vi "ForLoopNotes.vi"() -> ()   [LabVIEW 2012]
panel:
  out "3 Loops Ago":dbl
  out "2 Loops Ago":dbl
  out "End Value":dbl
  out "New Value":dbl
  out "1 Loop Ago":dbl
  out "i":dbl
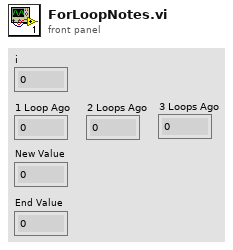
[diagram p1: front panel]
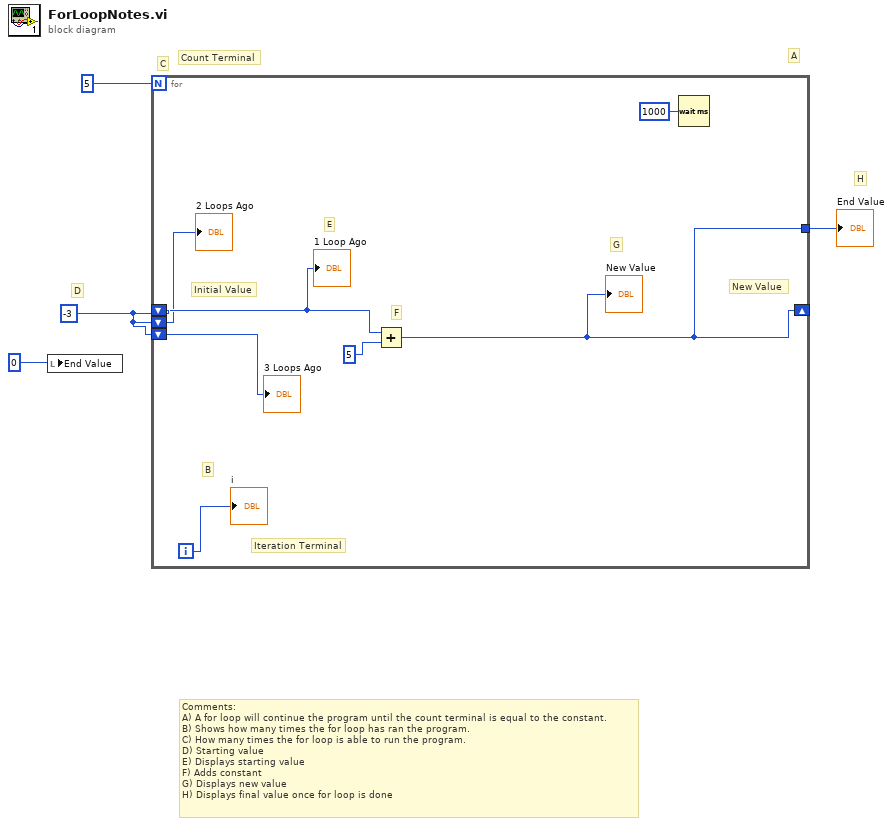
[diagram p0: block diagram]
diagram:
  w1 = -3
  # "H"
  # "D"
  # "C"
  # "Count Terminal"
  # "Comments:\nA) A for loop will continue the program until the count terminal is equal to the constant.\nB) Shows how many times the for loop has ran the program.\nC) How many times the for loop is able to run the program.\nD) Starting value\nE) Displays starting value\nF) Adds constant\nG) Displays new value\nH) Displays final value once for loop is done"
  # "A"
  n1 = local write "End Value"(0) -> ()
  n2 = for {
    N: 5 -> [_]
    shift-right: [w7] -> _
    shift-left: w1 -> [w8]
    tunnel: [w7] -> w3
    shift-left: w1 -> [w5]
    shift-left: w1 -> [w6]
    i -> [w9]
    # "G"
    # "F"
    # "E"
    # "B"
    # "New Value"
    # "Initial Value"
    # "Iteration Terminal"
    n3 = Add(x=w8, y=5) -> (x+y=w7:i32)
    "New Value" <- w7
    n4 = Wait (ms)(milliseconds to wait=u32 1000) -> ()  [unwired: 1 out]
    "i" <- w9
    "1 Loop Ago" <- w8
    "3 Loops Ago" <- w6
    "2 Loops Ago" <- w5
  }
  "End Value" <- w3
